vi "Decompose Map.vi"(8 "error in (no error)":errorcluster, 11 "Variant Map":variant) -> (0 "error out":errorcluster, 1 "Values":variant[](array[variant]), 2 "Keys":variant[](array[variant]), 3 "Size":i32)   [LabVIEW 2017, in "Composition.lvlib"]
doc: "Decomposes a Variant Map into keys and values. Maps are available in LabVIEW 2019 and higher."
uses:
  Composition.lvlib
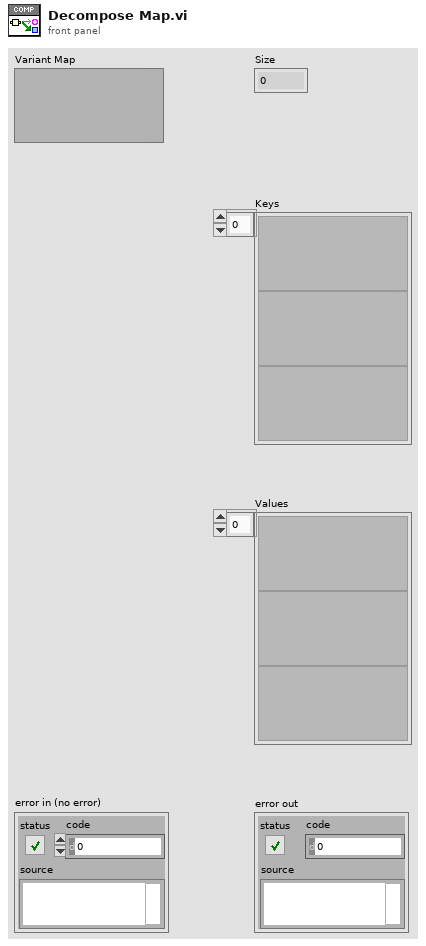
[diagram p1: front panel]
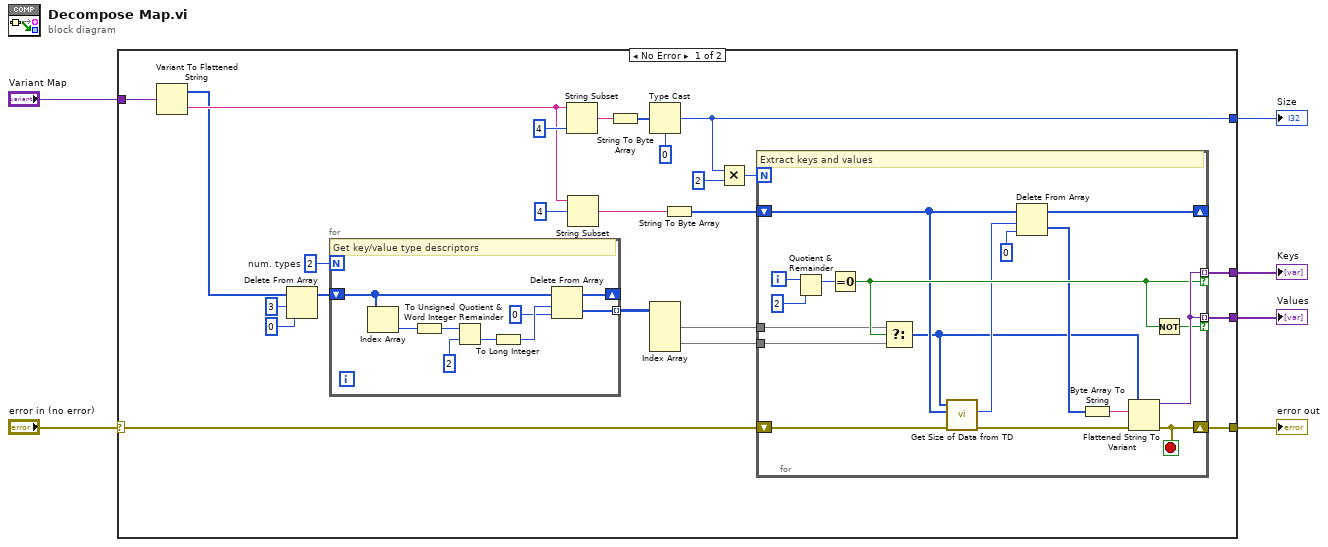
[diagram p0: block diagram]
diagram:
  n1 = case shown="No Error" "error in (no error)" {
    selector: "error in (no error)" -> [w18 w58]
    tunnel: [w23 _] -> w6
    tunnel: [w22 _] -> w5
    tunnel: "Variant Map" -> [w21 _]
    tunnel: [w20 w58] -> w3
    tunnel: [w19 _] -> w2
    frame No Error {
      w13 = 2  # num. types
      n2 = Variant To Flattened String(Variant=w21) -> (data string=w26:string, 1:w17:i16[])
      n3 = Delete From Array(array=w17, length=3, index=0) -> (array with subset deleted=w14:i16[])  [unwired: 1 out]
      n4 = for {
        N: w13 -> [_]
        shift-right: [w32] -> _
        shift-left: w14 -> [w39]
        tunnel: [w31] -> w12 mode=indexing
        # "Get key/value type descriptors"
        n5 = Index Array(array=w39) -> (element=w38:i16)  [unwired: 1 in]
        n6 = To Unsigned Word Integer(number=w38) -> (unsigned 16bit integer=w36:u16)
        n7 = Quotient & Remainder(x=w36, y=u16 2) -> (floor(x/y)=w35:u16)  [unwired: 1 out]
        n8 = To Long Integer(number=w35) -> (32bit integer=w34:i32)
        n9 = Delete From Array(array=w39, length=w34, index=0) -> (deleted portion=w31:i16[], array with subset deleted=w32:i16[])
      }
      n10 = String Subset(string=w26, length (rest)=4 ("length (rest)")) -> (substring=w30:string)  [unwired: 1 in]
      n11 = String Subset(string=w26, offset (0)=4) -> (substring=w24:string)  [unwired: 1 in]
      n12 = String To Byte Array(string=w30) -> (unsigned byte array=w27:u8[])
      n13 = Type Cast(type=0, x=w27) -> (*(type *) &x=w19:i32)
      n14 = Index Array(array=w12) -> (element #1=w11:i16[], element #2=w10:i16[])  [unwired: 4 in]
      n15 = String To Byte Array(string=w24) -> (unsigned byte array=w7:u8[])
      n16 = Multiply(x=w19, y=2 ("x")) -> (x*y=w9:i32)
      n17 = for {
        N: w9 -> [_]
        shift-right: [w47] -> _
        shift-left: w7 -> [w41]
        tunnel: w11 -> [w49]
        tunnel: w10 -> [w48]
        tunnel: [w54] -> w23 mode=indexing if=w53
        tunnel: [w54] -> w22 mode=indexing if=w52
        shift-right: [w50] -> w20
        shift-left: w18 -> [w44]
        i -> [w57]
        stop <- w50 stop-if-true
        # "Extract keys and values"
        n18 = Quotient & Remainder(x=w57, y=2) -> (x-y*floor(x/y)=w55:i32)  [unwired: 1 out]
        n19 = Equal To 0?(x=w55) -> (x = 0?=w53:bool)
        n20 = Select(t=w49, s=w53, f=w48) -> (s? t:f=w40:i16[])
        n21 = call "Get Size of Data from TD.vi"("error in (no error)"=w44, "Data String"=w41, "Type Descriptor"=w40) -> ("error out"=w43:errorcluster, "Size of Data"=w42:i32)  [unwired: 7 in]
        n22 = Delete From Array(array=w41, length=w42, index=0) -> (deleted portion=w45:u8[], array with subset deleted=w47:u8[])
        n23 = Byte Array To String(unsigned byte array=w45) -> (string=w51:string)
        n24 = Flattened String To Variant(4:w43, 6:w51, 7:w40) -> (0:w50:errorcluster, 3:w54:variant)
        n25 = Not(x=w53) -> (.not. x?=w52:bool)
      }
    }
    frame Error {
    }
  }
  "Size" <- w2
  "Keys" <- w6
  "Values" <- w5
  "error out" <- w3
